vi "Execute ECal.vi"(4 "Port 3  (3)":i32=3, 6 "Port 2  (2)":i32=2, 7 "Channel (1)":i32=1, 8 "error in (no error)":errorcluster, 9 "Port 1 (1)":i32=1, 10 "Calibration (0: 1-port)":u16(ring) items=["1-port", "Full 2-port", "Full 3-port", "Full 4-port", "Response", "Confidence Check", "Enhanced Response"], 11 "VISA resource name":refnum<visa-resource-name>) -> (0 "error out":errorcluster, 3 "VISA resource name out":refnum<visa-resource-name>)   [LabVIEW 2022 SP3, in "Agilent ENA Series.lvlib"]
doc: "Executes 1-port, full 2-port, full 3-port, full 4-port, response calibration or the confidence check of the specified ports of selected channel using the ECal (Electrical Calibration) module."
uses:
  <instrlib>/Agilent ENA Series/Agilent ENA Series.lvlib
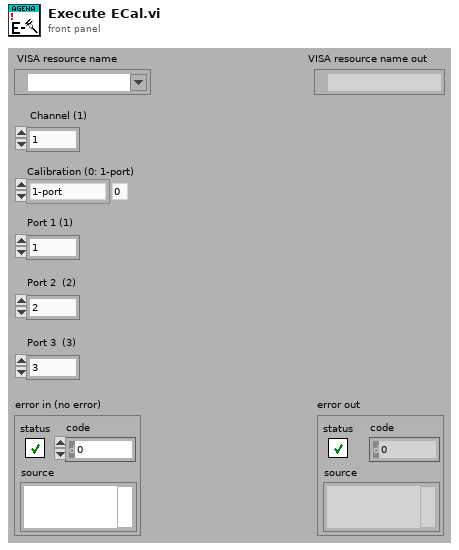
[diagram p1: front panel]
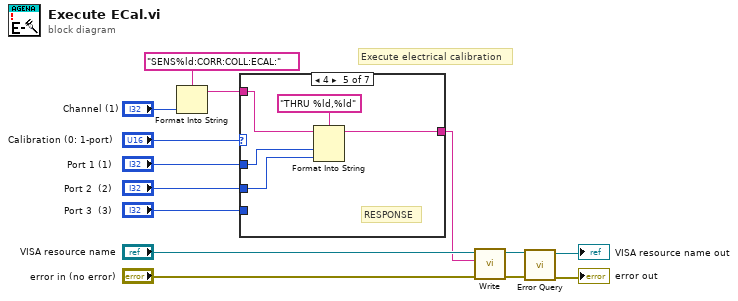
[diagram p0: block diagram]
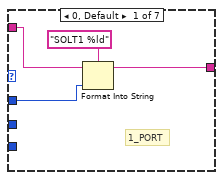
[diagram p2: hidden frame]
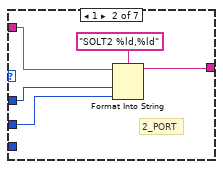
[diagram p3: hidden frame]
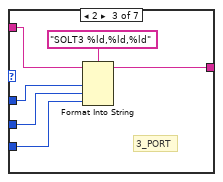
[diagram p4: hidden frame]
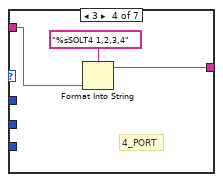
[diagram p5: hidden frame]
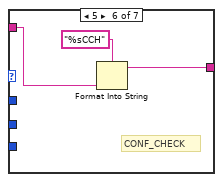
[diagram p6: hidden frame]
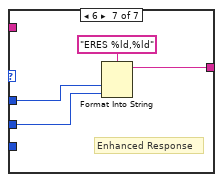
[diagram p7: hidden frame]
diagram:
  # "Execute electrical calibration"
  n1 = Format Into String(format string="SENS%ld:CORR:COLL:ECAL:", "Channel (1)") -> (resulting string=w8:string)  [unwired: 2 in, 1 out]
  n2 = case shown="4" "Calibration (0: 1-port)" {
    tunnel: "Port 1 (1)" -> [w17 w21 w28 _ w36 _ w43]
    tunnel: w8 -> [w16 w22 w27 w30 w35 w39 _]
    tunnel: [w15 w19 w26 w31 w34 w38 w41] -> w5
    tunnel: "Port 2  (2)" -> [_ w20 w25 _ w33 _ w42]
    tunnel: "Port 3  (3)" -> [_ _ w24 _ _ _ _]
    frame 0, Default {
      # "1_PORT"
      n3 = Format Into String(format string="SOLT1 %ld", initial string=w16, w17) -> (resulting string=w15:string)  [unwired: 1 in, 1 out]
    }
    frame 1 {
      # "2_PORT"
      n4 = Format Into String(format string="SOLT2 %ld,%ld", initial string=w22, w21, w20) -> (resulting string=w19:string)  [unwired: 1 in, 1 out]
    }
    frame 2 {
      # "3_PORT"
      n5 = Format Into String(format string="SOLT3 %ld,%ld,%ld", initial string=w27, w28, w25, w24) -> (resulting string=w26:string)  [unwired: 1 in, 1 out]
    }
    frame 3 {
      # "4_PORT"
      n6 = Format Into String(format string="%sSOLT4 1,2,3,4", w30) -> (resulting string=w31:string)  [unwired: 2 in, 1 out]
    }
    frame 4 {
      # "RESPONSE"
      n7 = Format Into String(format string="THRU %ld,%ld", initial string=w35, w36, w33) -> (resulting string=w34:string)  [unwired: 1 in, 1 out]
    }
    frame 5 {
      # "CONF_CHECK"
      n8 = Format Into String(format string="%sCCH", w39) -> (resulting string=w38:string)  [unwired: 2 in, 1 out]
    }
    frame 6 {
      # "Enhanced Response"
      n9 = Format Into String(format string="ERES %ld,%ld", w43, w42) -> (resulting string=w41:string)  [unwired: 2 in, 1 out]
    }
  }
  n10 = call <instrlib>:"Write.vi"("error in (no error)"="error in (no error)", "String ()"=w5, "VISA resource name"="VISA resource name") -> ("error out"=w3:errorcluster, "VISA resource name out"=w4:refnum<visa-resource-name>)  [unwired: 6 in, 1 out]
  n11 = call <instrlib>:"Error Query.vi"("error in (no error)"=w3, "VISA resource name"=w4) -> ("error out"=→"error out":errorcluster, "VISA resource name out"=→"VISA resource name out":refnum<visa-resource-name>)  [unwired: 6 in, 2 out]
